vi "AddStaircasePotentialVoltammetry.vi"(0 "deviceName":string, 1 "channel":u8, 2 "repeats":u16=1, 3 "quietTime":sgl, 4 "quietTimeSamplingInterval":sgl=1.0, 5 "startVoltage":sgl, 6 "isStartVoltageVsOCP":bool, 7 "error in (no error)":errorcluster, 8 "endVoltage":sgl, 9 "isEndVoltageVsOCP":bool, 10 "firstVoltageLimit":sgl, 11 "isFirstVoltageLimitVsOCP":bool, 12 "secondVoltageLimit":sgl, 13 "isSecondVoltageLimitVsOCP":bool, 14 "stepSize":sgl, 15 "stepDuration":sgl, 16 "samplingInterval":sgl, 17 "approxMaxCurrent":sgl=inf, 18 "isAutorange":bool=TRUE, 19 "numberOfCycles":u32=1) -> (27 "error out":errorcluster)   [LabVIEW 2018]
doc: "EXPORT void AisAddStaircasePotentialVoltammetry(const char* deviceName, uint8_t channel, uint16_t repeats, float quietTime, float quietTimeSamplingInterval, float startVoltage, bool isStartVoltageVsOCP, float endVoltage, bool isEndVoltageVsOCP, float firstVoltageLimit, bool isFirstVoltageLimitVsOCP, float secondVoltageLimit, bool isSecondVoltageLimitVsOCP, float stepSize, float stepDuration, float samplingInterval, float approxMaxCurrent, bool isAutorange, unsigned int numberOfCycles);"
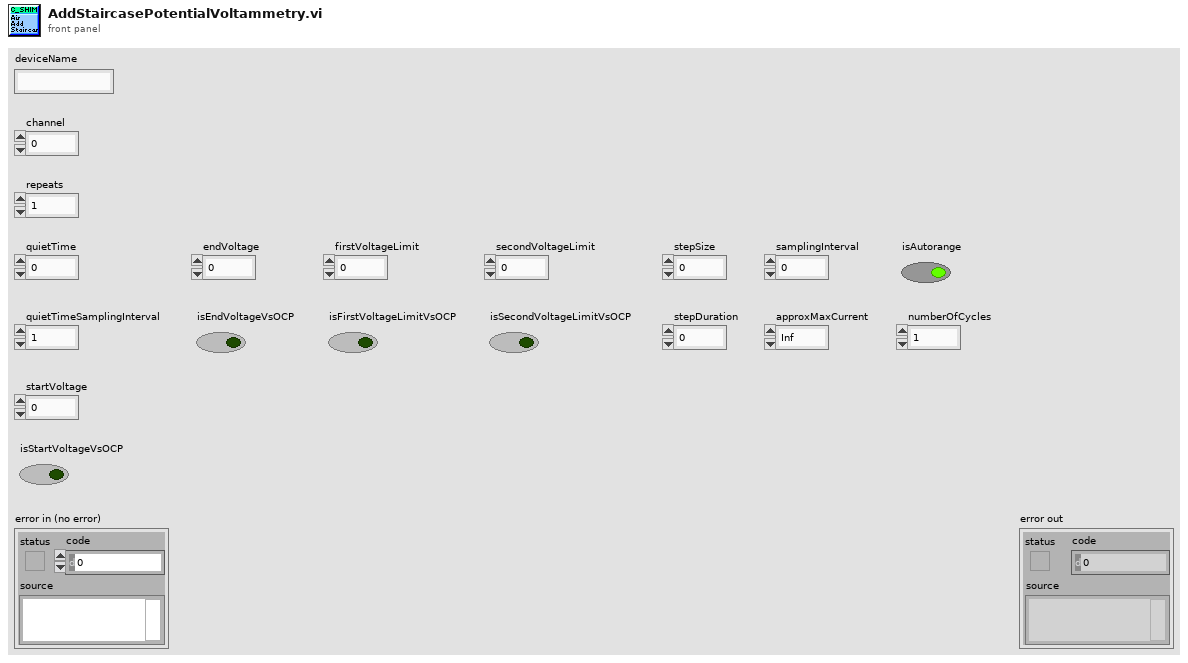
[diagram p1: front panel]
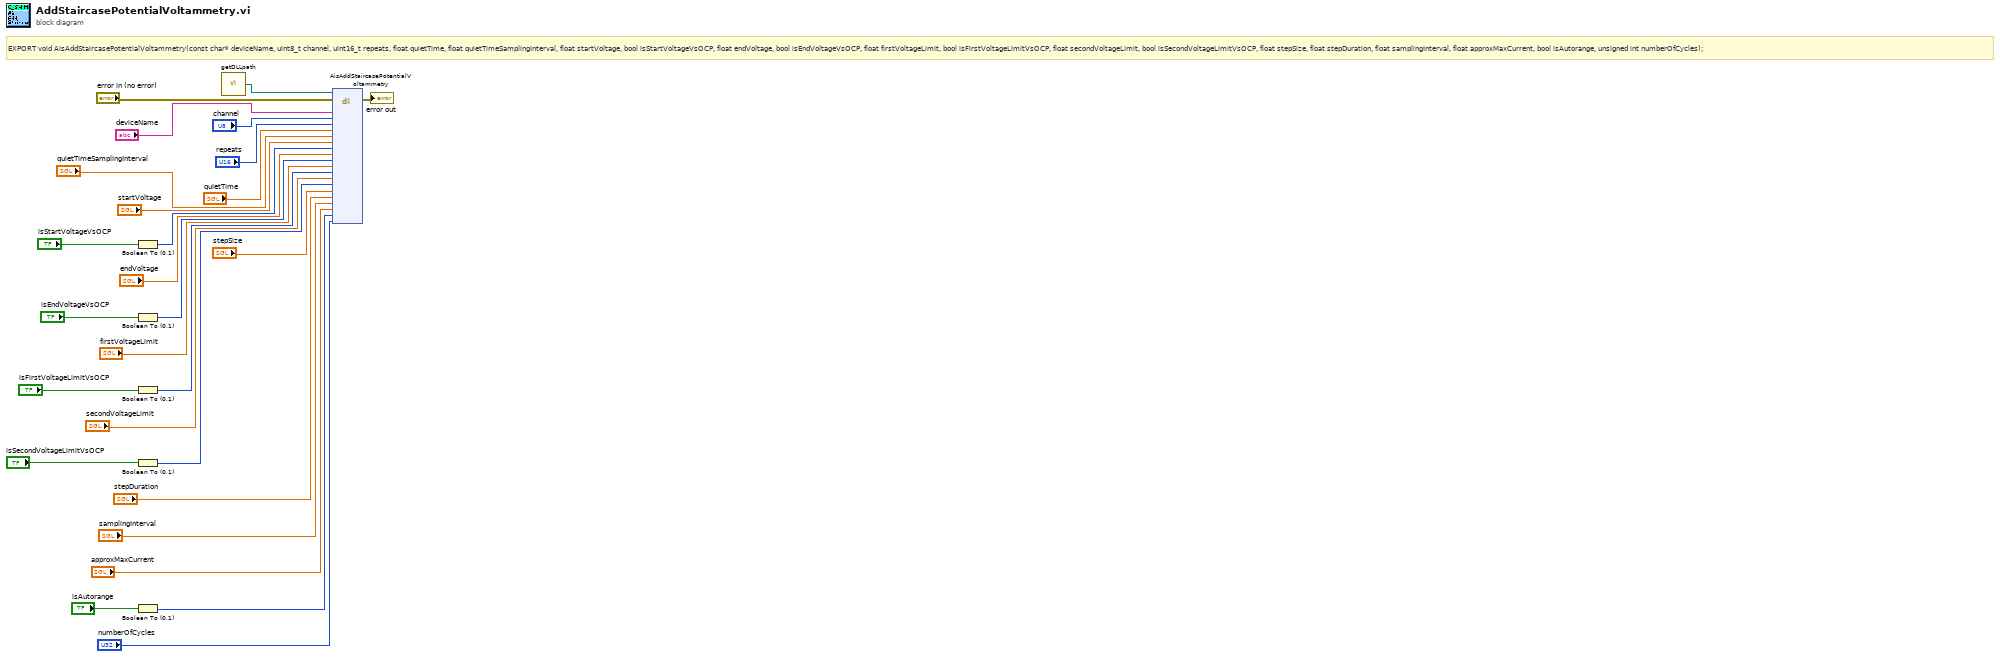
[diagram p0: block diagram]
diagram:
  # "EXPORT void AisAddStaircasePotentialVoltammetry(const char* deviceName, uint8_t channel, uint16_t repeats, float quietTime, float quietTimeSamplingInterval, float startVoltage, bool isStartVoltageVsOCP, float endVoltage, bool isEndVoltageVsOCP, float firstVoltageLimit, bool isFirstVoltageLimitVsOCP, float secondVoltageLimit, bool isSecondVoltageLimitVsOCP, float stepSize, float stepDuration, float samplingInterval, float approxMaxCurrent, bool isAutorange, unsigned int numberOfCycles);"
  n1 = Boolean To (0,1)(Boolean="isStartVoltageVsOCP") -> (0, 1=w20:i16)
  n2 = Boolean To (0,1)(Boolean="isEndVoltageVsOCP") -> (0, 1=w17:i16)
  n3 = Boolean To (0,1)(Boolean="isFirstVoltageLimitVsOCP") -> (0, 1=w14:i16)
  n4 = Boolean To (0,1)(Boolean="isSecondVoltageLimitVsOCP") -> (0, 1=w11:i16)
  n5 = Boolean To (0,1)(Boolean="isAutorange") -> (0, 1=w5:i16)
  n6 = call "getDLLpath.vi"() -> ("DLL_Path"=w1:path)
  n7 = dll-call lib="?" fn="AisAddStaircasePotentialVoltammetry"(path in=w1, error in="error in (no error)", "deviceName"="deviceName", "channel"="channel", "repeats"="repeats", "quietTime"="quietTime", "quietTimeSamplingInterval"="quietTimeSamplingInterval", "startVoltage"="startVoltage", "isStartVoltageVsOCP"=w20, "endVoltage"="endVoltage", "isEndVoltageVsOCP"=w17, "firstVoltageLimit"="firstVoltageLimit", "isFirstVoltageLimitVsOCP"=w14, "secondVoltageLimit"="secondVoltageLimit", "isSecondVoltageLimitVsOCP"=w11, "stepSize"="stepSize", "stepDuration"="stepDuration", "samplingInterval"="samplingInterval", "approxMaxCurrent"="approxMaxCurrent", "isAutorange"=w5, "numberOfCycles"="numberOfCycles") -> (error out=→"error out":errorcluster)  [unwired: 21 in, 1 out]
